vi "Flatten welding results.vi"(0 "welding results":string) -> (4 "welding results  cluster":T1)   [LabVIEW 2020, in "ultrasonic welding machine.lvlib"]
uses:
  ultrasonic welding machine.lvlib
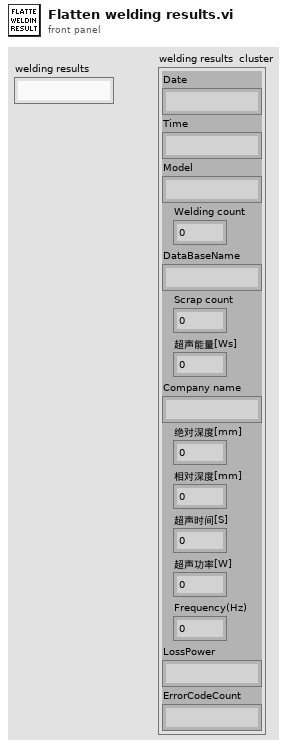
[diagram p1: front panel]
types:
  T1 = cluster{"Date":string, "Time":string, "Model":string, "Welding count ":i32, "DataBaseName":string, "Scrap count ":i32, "超声能量[Ws]":dbl, "Company name ":string, "绝对深度[mm]":dbl, "相对深度[mm]":dbl, "超声时间[S]":dbl, "超声功率[W]":dbl, "Frequency(Hz)":dbl, "LossPower":string, "ErrorCodeCount":string}
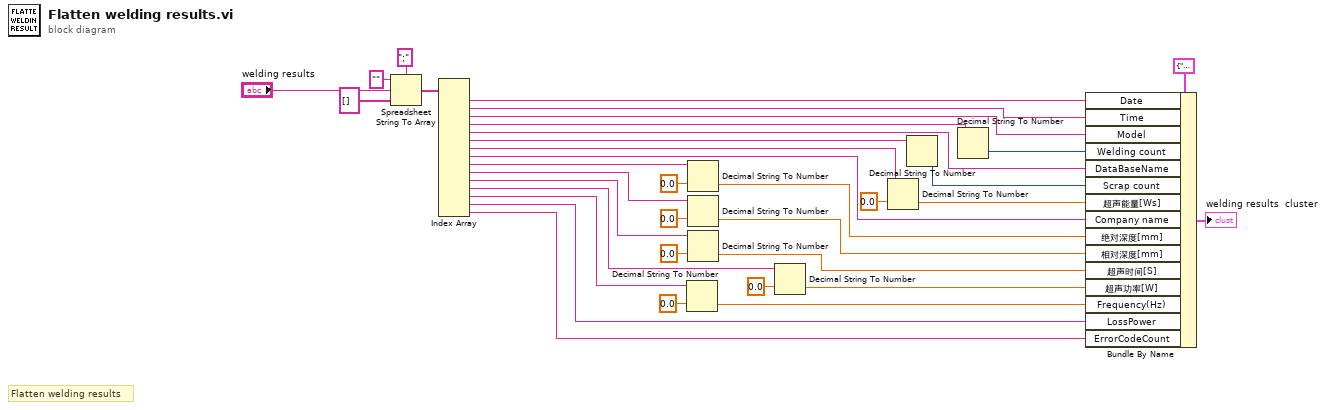
[diagram p0: block diagram]
diagram:
  # "Flatten welding results"
  n1 = Spreadsheet String To Array(delimiter (Tab)=";", format string="", spreadsheet string="welding results", array type (2D Dbl)=string[] []) -> (array=w5:string[])
  n2 = Index Array(array=w5) -> (element #1=w6:string, element #2=w7:string, element #3=w8:string, element #4=w9:string, element #5=w11:string, element #6=w12:string, element #7=w14:string, element #8=w16:string, element #9=w19:string, element #10=w21:string, element #11=w23:string, element #12=w29:string, element #13=w30:string, element #14=w33:string, element #15=w34:string)  [unwired: 15 in]
  n3 = Decimal String To Number(string=w30, default (0L)=0.0 ("绝对深度[mm]")) -> (number=w32:dbl)  [unwired: 1 in, 1 out]
  n4 = Decimal String To Number(string=w19, default (0L)=0.0 ("绝对深度[mm]")) -> (number=w24:dbl)  [unwired: 1 in, 1 out]
  n5 = Decimal String To Number(string=w21, default (0L)=0.0 ("绝对深度[mm]")) -> (number=w25:dbl)  [unwired: 1 in, 1 out]
  n6 = Decimal String To Number(string=w23, default (0L)=0.0 ("绝对深度[mm]")) -> (number=w26:dbl)  [unwired: 1 in, 1 out]
  n7 = Decimal String To Number(string=w29, default (0L)=0.0 ("绝对深度[mm]")) -> (number=w31:dbl)  [unwired: 1 in, 1 out]
  n8 = Decimal String To Number(string=w14, default (0L)=0.0 ("绝对深度[mm]")) -> (number=w15:dbl)  [unwired: 1 in, 1 out]
  n9 = Decimal String To Number(string=w12) -> (number=w13:i32)  [unwired: 2 in, 1 out]
  n10 = Decimal String To Number(string=w9) -> (number=w10:i32)  [unwired: 2 in, 1 out]
  n11 = Bundle By Name(cluster=T1 {"Date"="", "Time"="", "Model"="", "Welding count "=0, "DataBaseName"="", "Scrap count "=0, "超声能量[Ws]"=0.0, "Company name "="", "绝对深度[mm]"=0.0, "相对深度[mm]"=0.0, "超声时间[S]"=0.0, "超声功率[W]"=0.0, "Frequency(Hz)"=0.0, "LossPower"="", "ErrorCodeCount"=""}, "Date"=w6, "Time"=w7, "Model"=w8, "Welding count"=w10, "DataBaseName"=w11, "Scrap count"=w13, "超声能量[Ws]"=w15, "Company name"=w16, "绝对深度[mm]"=w24, "相对深度[mm]"=w25, "超声时间[S]"=w26, "超声功率[W]"=w31, "Frequency(Hz)"=w32, "LossPower"=w33, "ErrorCodeCount"=w34) -> (→"welding results  cluster":T1)
